vi "DisplayImage.vi"(0 "image color":T2, 1 "Array":u32[](array[numeric]), 3 "data type":T4(ring), 5 "Image grayscale":T2, 9 "width":u16, 11 "error in (no error)":errorcluster, 12 "height":u16, 13 "interpretation":T3(ring), 14 "bayer parameters":T1) -> (4 "display image":T2, 15 "error out":errorcluster)   [LabVIEW 2025]
uses:
  <vilib>/vision/Image Controls.llb/IMAQ Image.ctl
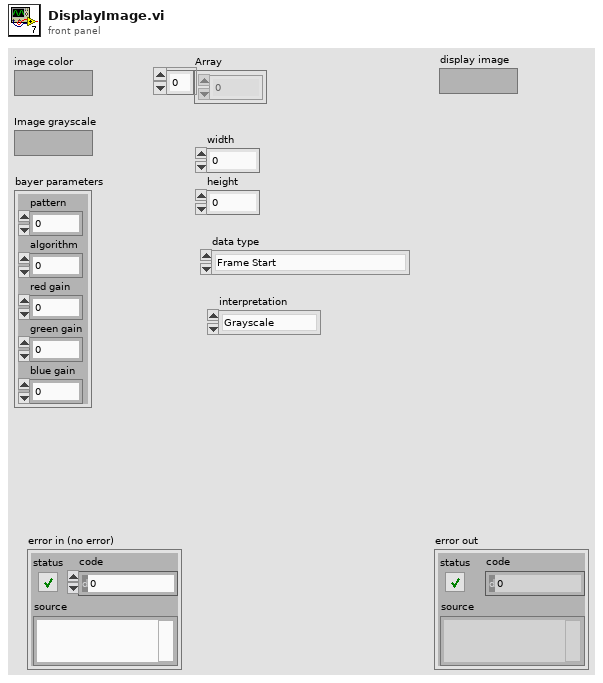
[diagram p1: front panel]
types:
  T1 = cluster{"pattern":i32, "algorithm":i32, "red gain":dbl, "green gain":dbl, "blue gain":dbl}
  T2 = typedef "IMAQ Image.ctl" = refnum<image>
  T3 = enum16{"Grayscale", "Bayer", "RGB", "YUV422", "YUV420", "Legacy YUV420"}
  T4 = enum8{"Frame Start", "Frame End", "Line Start", "Line End", "End of Transmission", "Reserved 0", "Reserved 1", "Reserved 2", "Generic Short Packet 1", "Generic Short Packet 2", "Generic Short Packet 3", "Generic Short Packet 4", "Generic Short Packet 5", "Generic Short Packet 6", "Generic Short Packet 7", "Generic Short Packet 8", "Null", "Blanking Data", "Embedded 8-bit non Image Data", "Generic Long Packet 1", "Generic Long Packet 2", "Generic Long Packet 3", "Generic Long Packet 4", "Reserved 3", "YUV420 8-bit", "YUV420 10-bit", "Legacy YUV420 8-bit", "Reserved 4", "YUV420 8-bit Chroma Shifted", "YUV420 10-bit Chroma Shifted", "YUV422 8-bit", "YUV422 10-bit", "RGB444", "RGB555", "RGB565", "RGB666", "RGB888", "Reserved 5", "Reserved 6", "RAW 24", "RAW 6", "RAW 7", "RAW 8", "RAW 10", "RAW 12", "RAW 14", "RAW 16", "RAW 20", "User Defined 8-bit Data 1", "User Defined 8-bit Data 2", "User Defined 8-bit Data 3", "User Defined 8-bit Data 4", "User Defined 8-bit Data 5", "User Defined 8-bit Data 6", "User Defined 8-bit Data 7", "User Defined 8-bit Data 8", "USL Command", "Reserved 7", "Reserved 8", "Reserved 9", "Reserved 10", "Reserved 11", "Reserved 12", "LRTE EPD Spacer"}
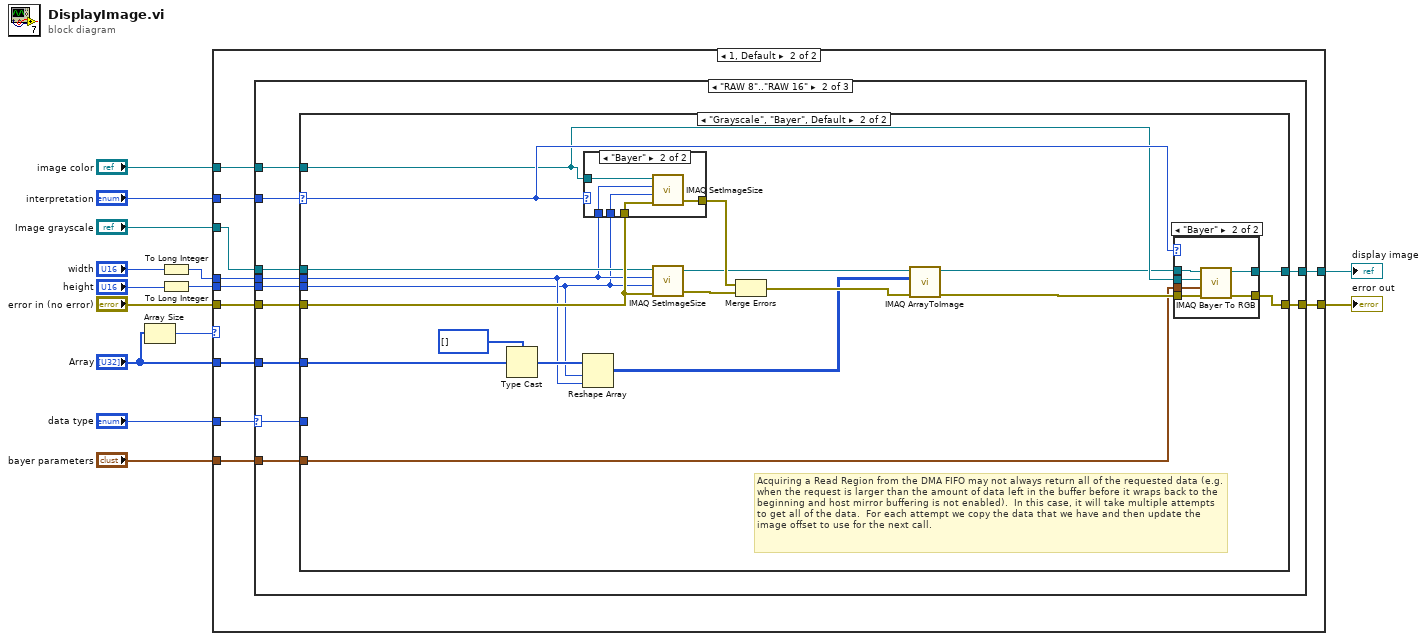
[diagram p0: block diagram]
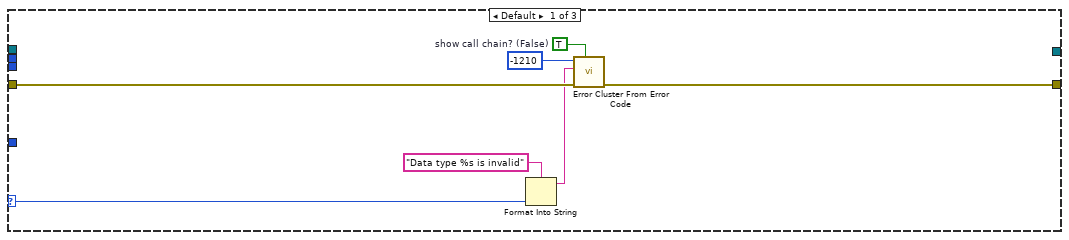
[diagram p3: hidden frame]
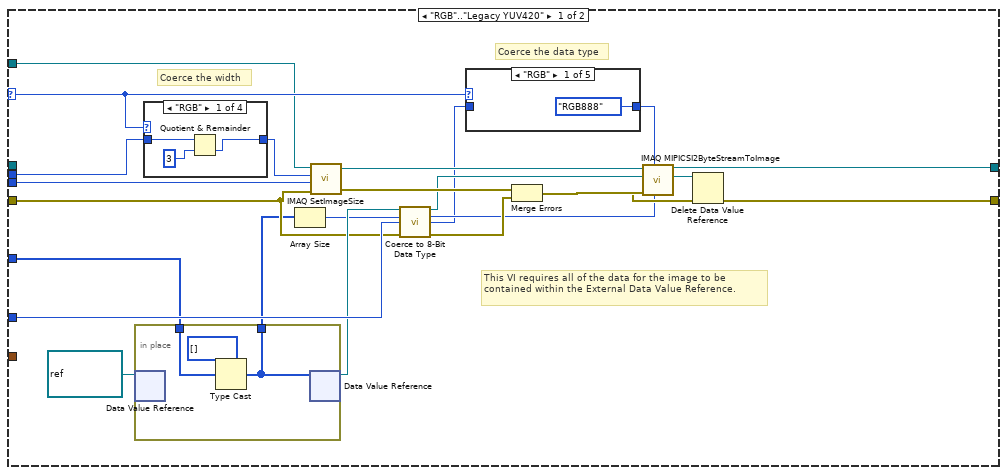
[diagram p4: hidden frame]
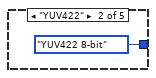
[diagram p5: hidden frame]
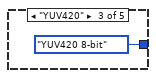
[diagram p6: hidden frame]
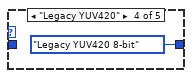
[diagram p7: hidden frame]
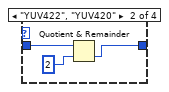
[diagram p9: hidden frame]
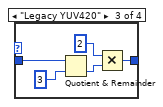
[diagram p10: hidden frame]
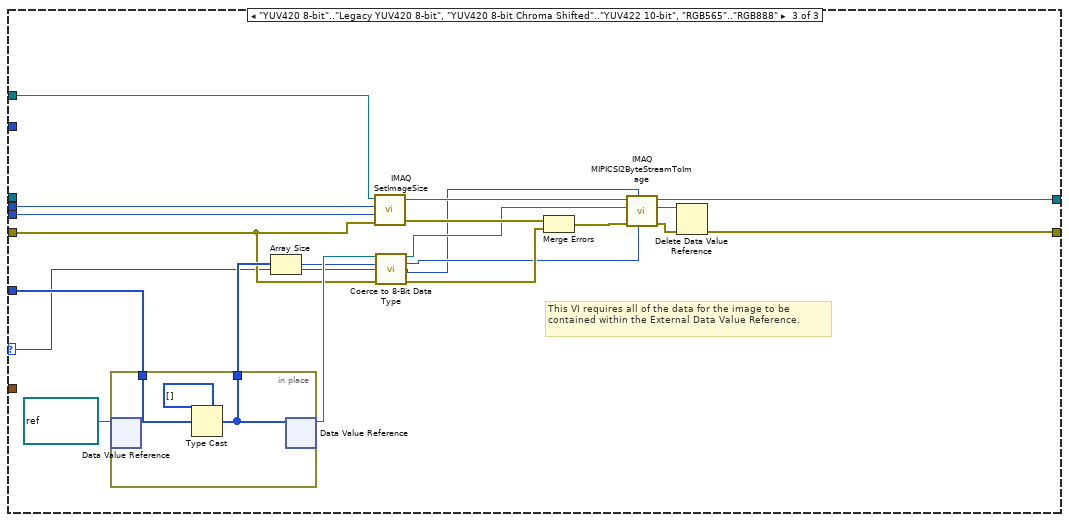
[diagram p14: hidden frame]
diagram:
  n1 = Array Size(array="Array") -> (size(s)=w1:i32)
  n2 = To Long Integer(number="width") -> (32bit integer=w12:i32)
  n3 = To Long Integer(number="height") -> (32bit integer=w13:i32)
  n4 = case shown="1, Default" w1 {
    tunnel: "error in (no error)" -> [w15 w27]
    tunnel: w13 -> [_ w26]
    tunnel: w12 -> [_ w25]
    tunnel: [w16 w24] -> w11
    tunnel: [w15 w23] -> w10
    tunnel: "data type" -> [_ w22]
    tunnel: "interpretation" -> [_ w21]
    tunnel: "image color" -> [_ w20]
    tunnel: "Image grayscale" -> [w16 w19]
    tunnel: "Array" -> [_ w18]
    tunnel: "bayer parameters" -> [_ w17]
    frame 0 {
    }
    frame 1, Default {
      n5 = case shown="\"RAW 8\"..\"RAW 16\"" w22 {
        selector: w22 -> [w28 w37 w126]
        tunnel: w27 -> [w32 w45 w130]
        tunnel: w26 -> [_ w44 w143]
        tunnel: w25 -> [_ w43 w142]
        tunnel: [_ w42 w138] -> w24
        tunnel: [w31 w41 w135] -> w23
        tunnel: w21 -> [_ w40 _]
        tunnel: w20 -> [_ w39 w124]
        tunnel: w19 -> [_ w38 _]
        tunnel: w18 -> [_ w36 w129]
        tunnel: w17 -> [_ w35 _]
        frame Default {
          w33 = TRUE  # show call chain? (False)
          n6 = Format Into String(format string="Data type %s is invalid" ("error message (\"\")"), w28) -> (resulting string=w29:string)  [unwired: 2 in, 1 out]
          n7 = call <vilib>:"Error Cluster From Error Code.vi"("show call chain? (False)"=w33, "error in (no error)"=w32, "error message (\"\")"=w29, "error code (0)"=-1210) -> ("error out"=w31:errorcluster)  [unwired: 5 in]
        }
        frame "RAW 8".."RAW 16" {
          n8 = case shown="\"Grayscale\", \"Bayer\", Default" w40 {
            selector: w40 -> [w56 w103]
            tunnel: w45 -> [w48 w107]
            tunnel: w44 -> [w59 w90]
            tunnel: w43 -> [w58 w91]
            tunnel: [w60 w105] -> w42
            tunnel: [w61 w104] -> w41
            tunnel: w39 -> [w53 w101]
            tunnel: w38 -> [_ w102]
            tunnel: w37 -> [w52 _]
            tunnel: w36 -> [w47 w94]
            tunnel: w35 -> [_ w92]
            frame "RGB".."Legacy YUV420" {
              # "Coerce the data type"
              # "Coerce the width"
              # "This VI requires all of the data for the image to be contained within the External Data Value Reference."
              n9 = in-place {
                in-place-border: w47 -> [w72]
                in-place-border: [w70] -> w46
                n10 = in-place-dvr #1(refnum<data-value> refnum ("image pixel data region")) -> ()  [unwired: 2 out]
                n11 = Type Cast(type=u8[] [], x=w72) -> (*(type *) &x=w70:u8[])
                n12 = in-place-dvr #1(w70) -> (w51:refnum<data-value>)  [unwired: 1 out]
              }
              n13 = case shown="\"RGB\"" w56 {
                tunnel: w58 -> [w79 w82 w88 w89]
                tunnel: [w78 w81 w85 w89] -> w57
                frame "RGB" {
                  n14 = Quotient & Remainder(x=w79, y=3) -> (floor(x/y)=w78:i32)  [unwired: 1 out]
                }
                frame "YUV422", "YUV420" {
                  n15 = Quotient & Remainder(x=w82, y=2) -> (floor(x/y)=w81:i32)  [unwired: 1 out]
                }
                frame "Legacy YUV420" {
                  n16 = Quotient & Remainder(x=w88, y=3) -> (floor(x/y)=w86:i32)  [unwired: 1 out]
                  n17 = Multiply(x=2, y=w86) -> (x*y=w85:i32)
                }
                frame Default {
                }
              }
              n18 = Array Size(array=w46) -> (size(s)=w49:i32)
              n19 = call "IMAQ SetImageSize"("error in (no error)"=w48, "Y Resolution"=w59, "X Resolution"=w57, "Image"=w53) -> ("error out"=w68:errorcluster, "Image Out"=w69:T2)  [unwired: 1 in]
              n20 = call "Coerce to 8-Bit Data Type.vi"("image pixel data region in"=w51, "image bytes in"=w49, "data type in"=w52, "error in (no error)"=w48) -> ("image pixel data region out"=w62:refnum<data-value>, "image bytes out"=w63:u32, "data type out"=w54:T4, "error out"=w64:errorcluster)  [unwired: 8 in]
              n21 = case shown="\"RGB\"" w56 {
                tunnel: w54 -> [_ _ _ _ w77]
                tunnel: [T4."RGB888" ("data type") T4."YUV422 8-bit" ("data type") T4."YUV420 8-bit" ("data type") T4."Legacy YUV420 8-bit" ("data type") w77] -> w55
                frame "RGB" {
                }
                frame "YUV422" {
                }
                frame "YUV420" {
                }
                frame "Legacy YUV420" {
                }
                frame Default {
                }
              }
              n22 = Merge Errors(w68, w64) -> (w67:errorcluster)
              n23 = call "IMAQ MIPICSI2ByteStreamToImage"("Bytes to Copy"=w63, "Format"=w55, "error in (no error)"=w67, "Byte Stream In"=w62, "Image In"=w69) -> ("error out"=w66:errorcluster, "Byte Stream Out"=w65:refnum<data-value>, "Image Out"=w60:T2)  [unwired: 3 in, 1 out]
              n24 = Delete Data Value Reference(data value reference=w65, error in=w66) -> (error out=w61:errorcluster)  [unwired: 1 out]
            }
            frame "Grayscale", "Bayer", Default {
              # "Acquiring a Read Region from the DMA FIFO may not always return all of the requested data (e.g. when the request is larger than the amount of data left in the buffer before it wraps back to the beginning and host mirror buffering is not enabled).  In this case, it will take multiple attempts to get all of the data.  For each attempt we copy the data that we have and then update the image offset to use for the next call."
              n25 = Type Cast(type=u8[] [], x=w94) -> (*(type *) &x=w95:u8[])
              n26 = Reshape Array(w95, w90, w91) -> (w93:u8[][])
              n27 = case shown="\"Bayer\"" w103 {
                tunnel: w107 -> [w109 w114]
                tunnel: [w109 w113] -> w106
                tunnel: w101 -> [_ w112]
                tunnel: w90 -> [_ w111]
                tunnel: w91 -> [_ w110]
                frame "Grayscale", Default {
                }
                frame "Bayer" {
                  n28 = call "IMAQ SetImageSize"("error in (no error)"=w114, "Y Resolution"=w111, "X Resolution"=w110, "Image"=w112) -> ("error out"=w113:errorcluster)  [unwired: 1 in, 1 out]
                }
              }
              n29 = call "IMAQ SetImageSize"("error in (no error)"=w107, "Y Resolution"=w90, "X Resolution"=w91, "Image"=w102) -> ("error out"=w108:errorcluster, "Image Out"=w100:T2)  [unwired: 1 in]
              n30 = Merge Errors(w106, w108) -> (w98:errorcluster)
              n31 = call "IMAQ ArrayToImage"("error in (no error)"=w98, "Image Pixels (U8)"=w93, "Image"=w100) -> ("error out"=w97:errorcluster, "Image Out"=w99:T2)  [unwired: 7 in]
              n32 = case shown="\"Bayer\"" w103 {
                tunnel: w99 -> [w115 w122]
                tunnel: [w115 w121] -> w105
                tunnel: w97 -> [w116 w120]
                tunnel: [w116 w119] -> w104
                tunnel: w101 -> [_ w118]
                tunnel: w92 -> [_ w117]
                frame "Grayscale", Default {
                }
                frame "Bayer" {
                  n33 = call "IMAQ Bayer To RGB"("error in (no error)"=w120, "Bayer Parameters"=w117, "Image Dst"=w118, "Image Src"=w122) -> ("error out"=w119:errorcluster, "Image Dst Out"=w121:T2)  [unwired: 6 in]
                }
              }
            }
          }
        }
        frame "YUV420 8-bit".."Legacy YUV420 8-bit", "YUV420 8-bit Chroma Shifted".."YUV422 10-bit", "RGB565".."RGB888" {
          # "This VI requires all of the data for the image to be contained within the External Data Value Reference."
          n34 = in-place {
            in-place-border: w129 -> [w146]
            in-place-border: [w144] -> w131
            n35 = in-place-dvr #2(refnum<data-value> refnum ("image pixel data region")) -> ()  [unwired: 2 out]
            n36 = Type Cast(type=u8[] [], x=w146) -> (*(type *) &x=w144:u8[])
            n37 = in-place-dvr #2(w144) -> (w134:refnum<data-value>)  [unwired: 1 out]
          }
          n38 = Array Size(array=w131) -> (size(s)=w132:i32)
          n39 = call "IMAQ SetImageSize"("error in (no error)"=w130, "Y Resolution"=w143, "X Resolution"=w142, "Image"=w124) -> ("error out"=w140:errorcluster, "Image Out"=w141:T2)  [unwired: 1 in]
          n40 = call "Coerce to 8-Bit Data Type.vi"("image pixel data region in"=w134, "image bytes in"=w132, "data type in"=w126, "error in (no error)"=w130) -> ("image pixel data region out"=w128:refnum<data-value>, "image bytes out"=w125:u32, "data type out"=w123:T4, "error out"=w127:errorcluster)  [unwired: 8 in]
          n41 = Merge Errors(w140, w127) -> (w139:errorcluster)
          n42 = call "IMAQ MIPICSI2ByteStreamToImage"("Bytes to Copy"=w125, "Format"=w123, "error in (no error)"=w139, "Byte Stream In"=w128, "Image In"=w141) -> ("error out"=w137:errorcluster, "Byte Stream Out"=w136:refnum<data-value>, "Image Out"=w138:T2)  [unwired: 3 in, 1 out]
          n43 = Delete Data Value Reference(data value reference=w136, error in=w137) -> (error out=w135:errorcluster)  [unwired: 1 out]
        }
      }
    }
  }
  "display image" <- w11
  "error out" <- w10
